vi "MongoDB.GetCollectionNames.vi"(8 "error in (no error)":errorcluster, 11 "MongoDB.Database in":refnum<class "MongoDB.Database.lvclass">) -> (0 "error out":errorcluster, 2 "CollectionNames":string[](array[string]), 3 "MongoDB.Database out":refnum<class "MongoDB.Database.lvclass">)   [LabVIEW 2014, in "MongoDB.Database.lvclass"]
uses:
  MongoDB.Database.lvclass
  MongoDB.Database.lvclass/MongoDB.Database.ctl
  C:/MongoData/Drivers/mongo-csharp-driver-2.0.0-beta4/mongo-csharp-driver-2.0.0-beta4/src/MongoDB.Driver.Legacy/bin/Release/MongoDB.Driver.Legacy.dll
  MongoData/Drivers/mongo-csharp-driver-2.0.0-beta4/mongo-csharp-driver-2.0.0-beta4/src/MongoDB.Driver.Legacy/bin/Release/MongoDB.Driver.Legacy.dll
panel:
  in  "GetCollectionNames":refnum<k24>
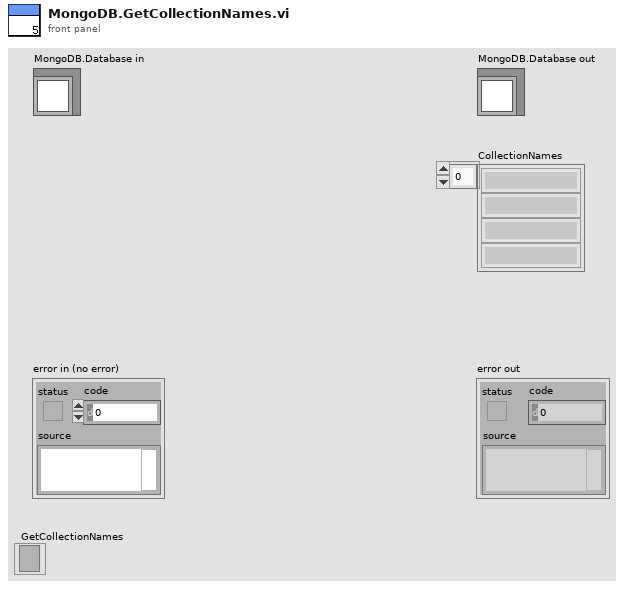
[diagram p1: front panel]
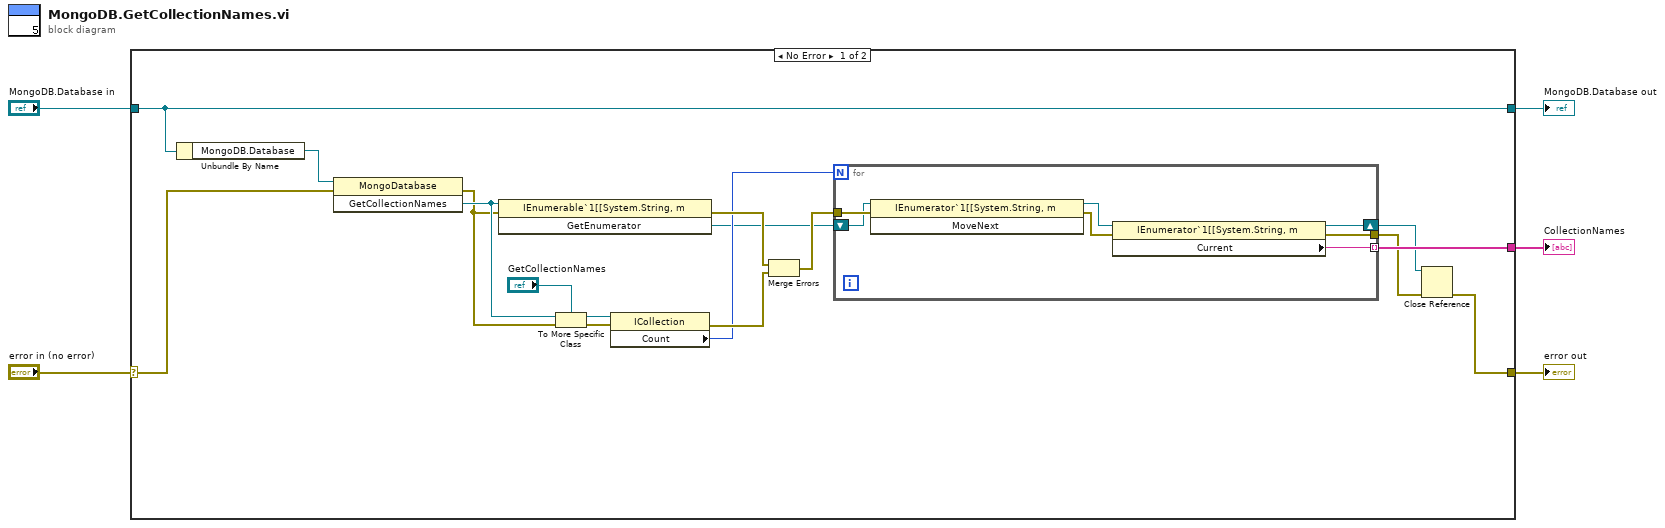
[diagram p0: block diagram]
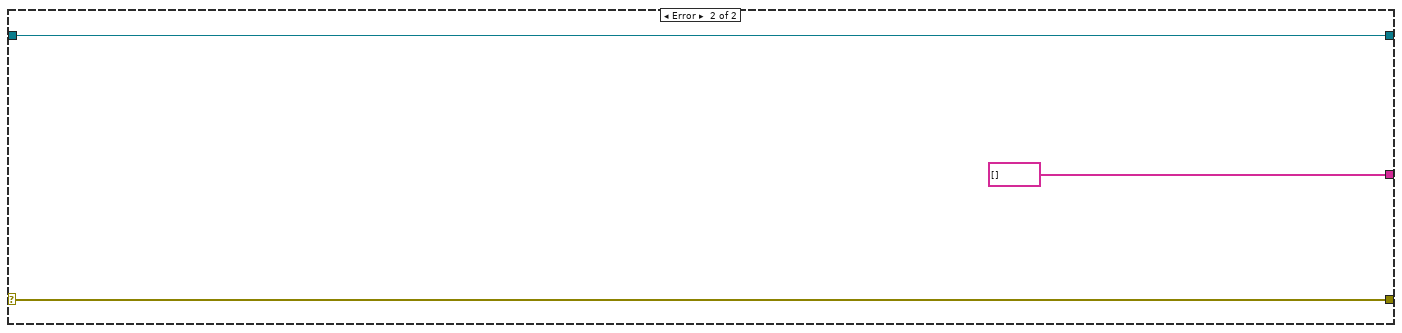
[diagram p2: hidden frame]
diagram:
  n1 = case shown="No Error" "error in (no error)" {
    selector: "error in (no error)" -> [w19 w32]
    tunnel: [w6 w32] -> w4
    tunnel: [w18 w31] -> w2
    tunnel: "MongoDB.Database in" -> [w18 w31]
    tunnel: [w9 string[] []] -> w1
    frame No Error {
      n2 = Unbundle By Name(w18) -> ("MongoDB.Database"=w17:refnum<k24>)
      n3 = invoke class="MongoDatabase" method="GetCollectionNames"(reference=w17, error in=w19) -> (error out=w12:errorcluster, "GetCollectionNames"=w20:refnum<k24>)  [unwired: 1 in, 1 out]
      n4 = invoke class="IEnumerable`1[[System.String, m" method="GetEnumerator"(reference=w20, error in=w12) -> (error out=w16:errorcluster, "GetEnumerator"=w10:refnum<k24>)  [unwired: 1 in, 1 out]
      n5 = To More Specific Class(target class="GetCollectionNames", reference=w20, error in=w12) -> (specific class reference=w21:refnum<k24>, error out=w13:errorcluster)
      n6 = property class="ICollection"(reference=w21, error in=w13) -> (error out=w15:errorcluster, "Count"=w11:i32)  [unwired: 1 out]
      n7 = Merge Errors(w16, w15) -> (w14:errorcluster)
      n8 = for {
        N: w11 -> [_]
        tunnel: w14 -> [w25]
        shift-right: [w28] -> w8
        shift-left: w10 -> [w23]
        tunnel: [w29] -> w9 mode=indexing
        tunnel: [w27] -> w7
        n9 = invoke class="IEnumerator`1[[System.String, m" method="MoveNext"(reference=w23, error in=w25) -> (reference out=w26:refnum<k24>, error out=w24:errorcluster)  [unwired: 1 in, 1 out]
        n10 = property class="IEnumerator`1[[System.String, m"(reference=w26, error in=w24) -> (reference out=w28:refnum<k24>, error out=w27:errorcluster, "Current"=w29:string)
      }
      n11 = Close Reference(reference=w8, error in (no error)=w7) -> (error out=w6:errorcluster)
    }
    frame Error {
    }
  }
  "error out" <- w4
  "MongoDB.Database out" <- w2
  "CollectionNames" <- w1
